vi "Build Messages.vi"(7 "Enumerations in":map{string, T1}(c390), 8 "error in (no error)":errorcluster, 9 "Messages in":map{string, T5}(c390), 10 "Segments in":T3[](array[typedef]), 11 "ProtoParser in":refnum<class "ProtoParser.lvclass">) -> (0 "error out":errorcluster, 1 "Messages":map{string, T5}(c390), 2 "Segments":T3[](array[typedef]), 3 "ProtoParser out":refnum<class "ProtoParser.lvclass">, 5 "Enumerations":map{string, T1}(c390))   [LabVIEW 2020, in "LV-Protoc.lvlib" / "ProtoParser.lvclass"]
uses:
  ProtoParser.lvclass
  Raw Segment.ctl
  Segment Type.ctl
  LV-Proto/Message.ctl
  LV-Proto/Field.ctl
  LV-Proto/Type.ctl
  LV-Proto/Proto Type.ctl
  LV-Proto/Enumeration.ctl
  LV-Proto/Enum Value.ctl
  LV-Protoc.lvlib
  LV-Proto/LV-Proto.lvlib
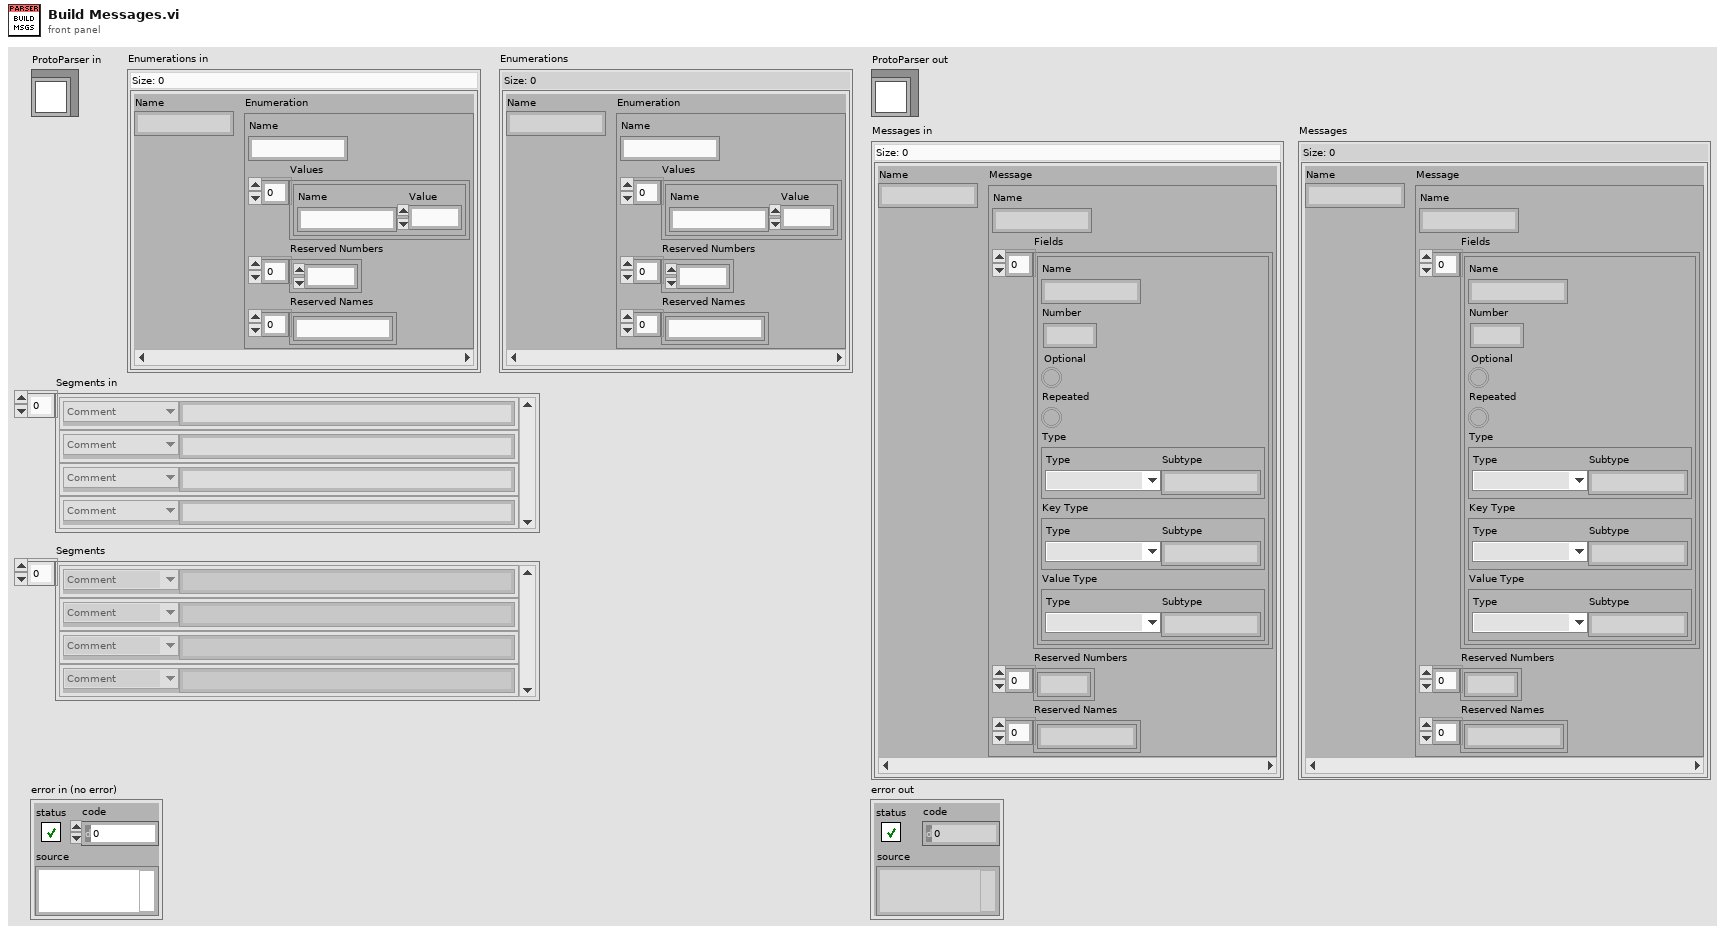
[diagram p1: front panel]
types:
  T1 = typedef "LV-Proto.lvlib/Enumeration.ctl" = cluster{"Name":string, "Values":T2[], "Reserved Numbers":u32[], "Reserved Names":string[]}
  T2 = typedef "LV-Proto.lvlib/Enum Value.ctl" = cluster{"Name":string, "Value":i32}
  T3 = typedef "LV-Protoc.lvlib/Raw Segment.ctl" = cluster{"Type":T4, "Text":string}
  T4 = typedef "LV-Protoc.lvlib/Segment Type.ctl" = enum16{"Comment", "Message Open", "Enum Open", "Message Close", "Enum Close", "Field", "Syntax", "Import", "Enum Value", "Package", "Reserved"}
  T5 = typedef "LV-Proto.lvlib/Message.ctl" = cluster{"Name":string, "Fields":T6[], "Reserved Numbers":u32[], "Reserved Names":string[]}
  T6 = typedef "LV-Proto.lvlib/Field.ctl" = cluster{"Name":string, "Number":u32, "Optional":bool, "Repeated":bool, "Type":T7, "Key Type":T7, "Value Type":T7}
  T7 = typedef "LV-Proto.lvlib/Type.ctl" = cluster{"Type":T8, "Subtype":string}
  T8 = typedef "LV-Proto.lvlib/Proto Type.ctl" = enum16{"UNKNOWN", "double", "float", "int32", "int64", "uint32", "uint64", "sint32", "sint64", "fixed32", "fixed64", "sfixed32", "sfixed64", "bool", "string", "bytes", "enum", "map", "message"}
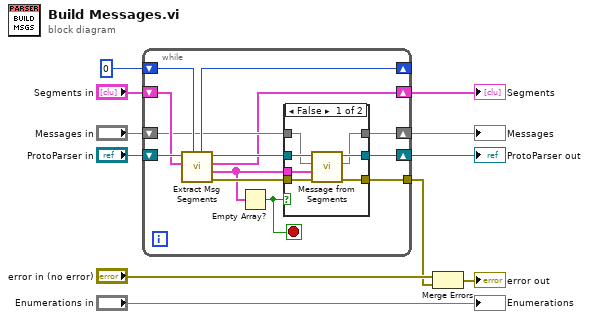
[diagram p0: block diagram]
diagram:
  n1 = while {
    shift-right: [w14] -> w6
    shift-left: "Segments in" -> [w22]
    shift-right: [w16] -> w3
    shift-left: "Messages in" -> [w17]
    shift-right: [w18] -> w7
    shift-left: "ProtoParser in" -> [w23]
    shift-right: [w19] -> _
    shift-left: 0 -> [w20]
    tunnel: [w12] -> w1
    stop <- w13 stop-if-true
    n2 = call "Extract Msg Segments.vi"("Start Index"=w20, "Segments in"=w22, "ProtoParser in"=w23) -> ("error out"=w24:errorcluster, "Message Segments"=w15:T3[], "Remaining"=w14:T3[], "ProtoParser out"=w21:refnum<class "ProtoParser.lvclass">, "Next Index"=w19:i32)  [unwired: 4 in]
    n3 = Empty Array?(array=w15) -> (empty?=w13:bool)
    n4 = case shown="False" w13 {
      tunnel: w21 -> [w31 w33]
      tunnel: [w27 w33] -> w18
      tunnel: w17 -> [w26 w34]
      tunnel: [w25 w34] -> w16
      tunnel: w15 -> [w30 _]
      tunnel: w24 -> [w29 w32]
      tunnel: [w28 w32] -> w12
      frame False {
        n5 = call "Message from Segments.vi"("error in (no error)"=w29, "Segments in"=w30, "Messages in"=w26, "ProtoParser in"=w31) -> ("error out"=w28:errorcluster, "Messages"=w25:map{string, T5}, "ProtoParser out"=w27:refnum<class "ProtoParser.lvclass">)  [unwired: 4 in, 1 out]
      }
      frame True {
      }
    }
  }
  "ProtoParser out" <- w7
  "Messages" <- w3
  "Segments" <- w6
  n6 = Merge Errors("error in (no error)", w1) -> (→"error out":errorcluster)
  "Enumerations" <- "Enumerations in"
